vi "WPI_CANTalonSRX_ChangeMode.vi"(6 "Master Device Number":u8, 8 "error in (no error)":errorcluster, 9 "Output":dbl, 10 "Control Mode":T1=enum."Unchanged / Invalid", 11 "CAN Talon SRX Ref":T2={"DeviceStatus"={"status"=FALSE, "code"=0, "source"=""}, "Type"=enum."PWM", "PWM"={"PWM Channel"=enum."PWM 1", "DeadBand"={"Name"="", "maxPositivePwm"=0, "minPositivePwm"=0, "centerPwm"=0, "maxNegativePwm"=0, "minNegativePwm"=0, "angularRange"=0}}, "CAN"={"Device Number"=0, "SetOutput VI Ref"=variant(enum8{"Percent VBus", "Current", "Speed", "Position", "Voltage"} enum."Percent VBus"), "GetOutput VI Ref"=variant(refnum<k1> refnum), "Enable VI Ref"=variant(dbl 12.0), "Disable VI Ref"=variant(enum8{"Percent VBus", "Speed", "Position", "Slave", "Unchanged / Invalid", "Voltage Compensation", "Current", "Motion Profile"} enum."Percent VBus"), "Data"=variant}, "Invert"=FALSE}) -> (0 "error out":errorcluster, 3 "CAN Talon SRX Ref":T2={"DeviceStatus"={"status"=FALSE, "code"=0, "source"=""}, "Type"=enum."PWM", "PWM"={"PWM Channel"=enum."PWM 1", "DeadBand"={"Name"="", "maxPositivePwm"=0, "minPositivePwm"=0, "centerPwm"=0, "maxNegativePwm"=0, "minNegativePwm"=0, "angularRange"=0}}, "CAN"={"Device Number"=0, "SetOutput VI Ref"=variant(enum8{"Percent VBus", "Current", "Speed", "Position", "Voltage"} enum."Percent VBus"), "GetOutput VI Ref"=variant(refnum<k1> refnum), "Enable VI Ref"=variant(dbl 12.0), "Disable VI Ref"=variant(enum8{"Percent VBus", "Speed", "Position", "Slave", "Unchanged / Invalid", "Voltage Compensation", "Current", "Motion Profile"} enum."Percent VBus"), "Data"=variant}, "Invert"=FALSE})   [LabVIEW 2016]
doc: "Changes the Control Mode of the Talon SRX.\n\nYou must also set the output value when changing the mode.\n\n<B>Master Device Number</B> is the CAN bus device ID of the master controller and must be set if placing the current Talon SRX into \"Slave\" mode."
uses:
  <vilib>/Rock Robotics/WPI/MotorControl/WPI_MotorControlDeviceRef.ctl
  <vilib>/Rock Robotics/WPI/MotorControl/WPI_MotorControlType.ctl
  <vilib>/Rock Robotics/SystemInterfaces/DIO/FPGA_DIOPWMChannel.ctl
  <vilib>/Rock Robotics/WPI/PWM/WPI_PWMDeadband.ctl
  <vilib>/Rock Robotics/WPI/ThirdParty/CanMotor/TalonSRX/WPI_CANTalonSRX_APIControlMode.ctl
  <vilib>/Rock Robotics/WPI/ThirdParty/CanMotor/TalonSRX/WPI_CANTalonSRX_GlobalOps.ctl
  <vilib>/Rock Robotics/WPI/ThirdParty/CanMotor/TalonSRX/CTRE_CANTalonSRX_UsageTypes.ctl
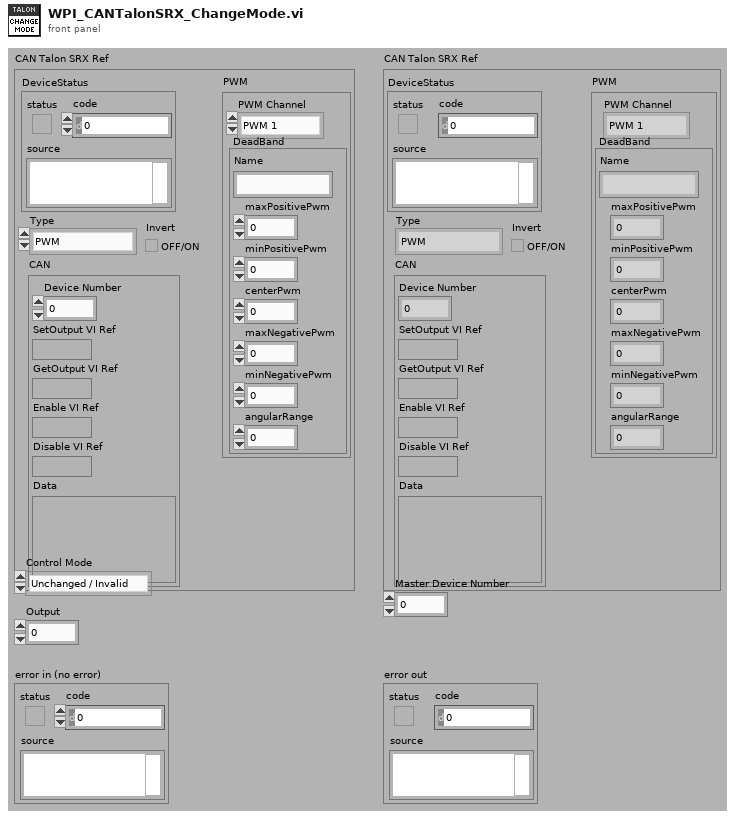
[diagram p1: front panel]
types:
  T1 = typedef "WPI_CANTalonSRX_APIControlMode.ctl" = enum8{"Percent VBus", "Speed", "Position", "Slave", "Unchanged / Invalid", "Voltage Compensation", "Current", "Motion Profile", "Motion Magic"}
  T2 = typedef "WPI_MotorControlDeviceRef.ctl" = cluster{"DeviceStatus":errorcluster, "Type":T3, "PWM":cluster{"PWM Channel":T4, "DeadBand":T5}, "CAN":cluster{"Device Number":u8, "SetOutput VI Ref":variant, "GetOutput VI Ref":variant, "Enable VI Ref":variant, "Disable VI Ref":variant, "Data":variant}, "Invert":bool}
  T3 = typedef "WPI_MotorControlType.ctl" = enum16{"PWM", "CAN"}
  T4 = typedef "FPGA_DIOPWMChannel.ctl" = enum8{"PWM 0", "PWM 1", "PWM 2", "PWM 3", "PWM 4", "PWM 5", "PWM 6", "PWM 7", "PWM 8", "PWM 9", "PWM MXP 0", "PWM MXP 1", "PWM MXP 2", "PWM MXP 3", "PWM MXP 4", "PWM MXP 5", "PWM MXP 6", "PWM MXP 7", "PWM MXP 8", "PWM MXP 9", "Invalid"}
  T5 = typedef "WPI_PWMDeadband.ctl" = cluster{"Name":string, "maxPositivePwm":i32, "minPositivePwm":i32, "centerPwm":i32, "maxNegativePwm":i32, "minNegativePwm":i32, "angularRange":u16}
  T6 = typedef "WPI_CANTalonSRX_GlobalOps.ctl" = enum16{"Read For Send", "Write After Receive General", "Write After Receive Feedback", "Write After Receive Encoder", "Write After Receive Ain", "Write Error", "Get All", "Set Output", "Set Mode", "Set Master ID", "Set Brake Mode", "Set Reverse Feedback Sensor", "Set Reverse Closed Loop Output", "Set Override Limits", "Set Forward Limit Enabled", "Set Reverse Limit Enabled", "Set Feedback Select", "Set Profile Select", "Set Throttle Ramp Rate", "Disable", "Set Enc Codes Per Rev", "Set Num Pot Turns", "Set Control Frame Rate", "Enable Legacy Control", "Write After Receive Pulse Width", "Set Enable Frame Rate", "Write After Receive Motion Profile", "Set Motion Profile Flow Control", "Set Motion Profile Control Frame Rate", "Set Current Limit Enable", "Set Usage Frame", "Write After Receive Motion Magic"}
  T7 = typedef "CTRE_CANTalonSRX_UsageTypes.ctl" = u32
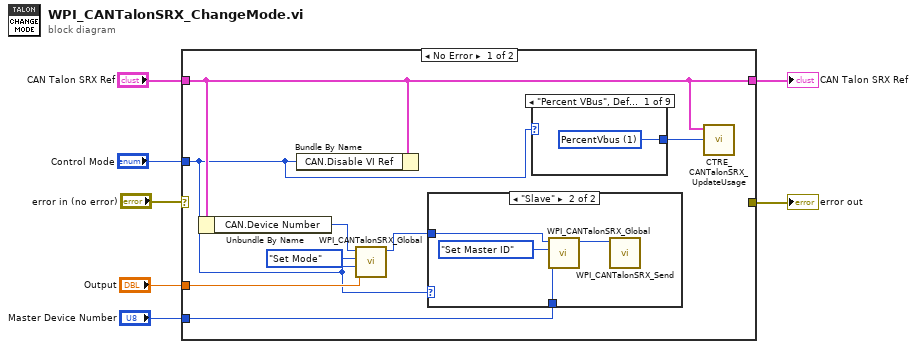
[diagram p0: block diagram]
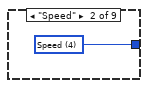
[diagram p2: hidden frame]
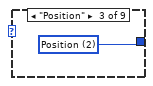
[diagram p3: hidden frame]
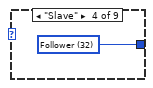
[diagram p4: hidden frame]
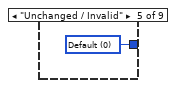
[diagram p5: hidden frame]
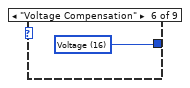
[diagram p6: hidden frame]
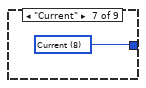
[diagram p7: hidden frame]
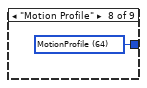
[diagram p8: hidden frame]
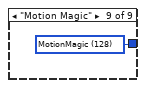
[diagram p9: hidden frame]
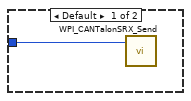
[diagram p10: hidden frame]
diagram:
  n1 = case shown="No Error" "error in (no error)" {
    selector: "error in (no error)" -> [_ w31]
    tunnel: [_ w31] -> w7
    tunnel: [w10 w30] -> w5
    tunnel: "CAN Talon SRX Ref" -> [w10 w30]
    tunnel: "Control Mode" -> [w8 _]
    tunnel: "Output" -> [w11 _]
    tunnel: "Master Device Number" -> [w12 _]
    frame No Error {
      n2 = Unbundle By Name(w10) -> ("CAN.Device Number"=w15:u8)
      n3 = Bundle By Name(cluster=w10, "CAN.Disable VI Ref"=w8) -> ()  [unwired: 1 out]
      n4 = call <vilib>:"WPI_CANTalonSRX_Global.vi"("Set Number"=w11, "Control Mode"=w8, "Operation"=WPI_CANTalonSRX_GlobalOps."Set Mode", "Device ID (0)"=w15) -> ("Device ID Out"=w13:u8)  [unwired: 5 in, 2 out]
      n5 = case shown="\"Slave\"" w8 {
        tunnel: w13 -> [w25 w28]
        tunnel: w12 -> [_ w27]
        frame Default {
          n6 = call <vilib>:"WPI_CANTalonSRX_Send.vi"("Device ID (0)"=w25) -> ()  [unwired: 10 in, 1 out]
        }
        frame "Slave" {
          n7 = call <vilib>:"WPI_CANTalonSRX_Global.vi"("Set Number"=w27, "Operation"=WPI_CANTalonSRX_GlobalOps."Set Master ID", "Device ID (0)"=w28) -> ("Device ID Out"=w26:u8)  [unwired: 6 in, 2 out]
          n8 = call <vilib>:"WPI_CANTalonSRX_Send.vi"("Device ID (0)"=w26) -> ()  [unwired: 10 in, 1 out]
        }
      }
      n9 = case shown="\"Percent VBus\", Default" w8 {
        tunnel: [w16 w17 w18 w19 w20 w21 w22 w23 w24] -> w9
        frame "Percent VBus", Default {
          w16 = T7 1 items=["Default"=0, "PercentVbus"=1, "Position"=2, "Speed"=4, "Current"=8, "Voltage"=16, "Follower"=32, "MotionProfile"=64, "MotionMagic"=128, "VRampRate"=4194304, "CurrentLimit"=8388608, "ZeroSensorI"=16777216, "ZeroSensorF"=33554432, "ZeroSensorR"=67108864, "ForwardLimitSwitch"=134217728, "ReverseLimitSwitch"=268435456, "ForwardSoftLimit"=536870912, "ReverseSoftLimit"=1073741824, "MultiProfile"=2147483648]
        }
        frame "Speed" {
          w17 = T7 4 items=["Default"=0, "PercentVbus"=1, "Position"=2, "Speed"=4, "Current"=8, "Voltage"=16, "Follower"=32, "MotionProfile"=64, "MotionMagic"=128, "VRampRate"=4194304, "CurrentLimit"=8388608, "ZeroSensorI"=16777216, "ZeroSensorF"=33554432, "ZeroSensorR"=67108864, "ForwardLimitSwitch"=134217728, "ReverseLimitSwitch"=268435456, "ForwardSoftLimit"=536870912, "ReverseSoftLimit"=1073741824, "MultiProfile"=2147483648]
        }
        frame "Position" {
          w18 = T7 2 items=["Default"=0, "PercentVbus"=1, "Position"=2, "Speed"=4, "Current"=8, "Voltage"=16, "Follower"=32, "MotionProfile"=64, "MotionMagic"=128, "VRampRate"=4194304, "CurrentLimit"=8388608, "ZeroSensorI"=16777216, "ZeroSensorF"=33554432, "ZeroSensorR"=67108864, "ForwardLimitSwitch"=134217728, "ReverseLimitSwitch"=268435456, "ForwardSoftLimit"=536870912, "ReverseSoftLimit"=1073741824, "MultiProfile"=2147483648]
        }
        frame "Slave" {
          w19 = T7 32 items=["Default"=0, "PercentVbus"=1, "Position"=2, "Speed"=4, "Current"=8, "Voltage"=16, "Follower"=32, "MotionProfile"=64, "MotionMagic"=128, "VRampRate"=4194304, "CurrentLimit"=8388608, "ZeroSensorI"=16777216, "ZeroSensorF"=33554432, "ZeroSensorR"=67108864, "ForwardLimitSwitch"=134217728, "ReverseLimitSwitch"=268435456, "ForwardSoftLimit"=536870912, "ReverseSoftLimit"=1073741824, "MultiProfile"=2147483648]
        }
        frame "Unchanged / Invalid" {
          w20 = T7 0 items=["Default"=0, "PercentVbus"=1, "Position"=2, "Speed"=4, "Current"=8, "Voltage"=16, "Follower"=32, "MotionProfile"=64, "MotionMagic"=128, "VRampRate"=4194304, "CurrentLimit"=8388608, "ZeroSensorI"=16777216, "ZeroSensorF"=33554432, "ZeroSensorR"=67108864, "ForwardLimitSwitch"=134217728, "ReverseLimitSwitch"=268435456, "ForwardSoftLimit"=536870912, "ReverseSoftLimit"=1073741824, "MultiProfile"=2147483648]
        }
        frame "Voltage Compensation" {
          w21 = T7 16 items=["Default"=0, "PercentVbus"=1, "Position"=2, "Speed"=4, "Current"=8, "Voltage"=16, "Follower"=32, "MotionProfile"=64, "MotionMagic"=128, "VRampRate"=4194304, "CurrentLimit"=8388608, "ZeroSensorI"=16777216, "ZeroSensorF"=33554432, "ZeroSensorR"=67108864, "ForwardLimitSwitch"=134217728, "ReverseLimitSwitch"=268435456, "ForwardSoftLimit"=536870912, "ReverseSoftLimit"=1073741824, "MultiProfile"=2147483648]
        }
        frame "Current" {
          w22 = T7 8 items=["Default"=0, "PercentVbus"=1, "Position"=2, "Speed"=4, "Current"=8, "Voltage"=16, "Follower"=32, "MotionProfile"=64, "MotionMagic"=128, "VRampRate"=4194304, "CurrentLimit"=8388608, "ZeroSensorI"=16777216, "ZeroSensorF"=33554432, "ZeroSensorR"=67108864, "ForwardLimitSwitch"=134217728, "ReverseLimitSwitch"=268435456, "ForwardSoftLimit"=536870912, "ReverseSoftLimit"=1073741824, "MultiProfile"=2147483648]
        }
        frame "Motion Profile" {
          w23 = T7 64 items=["Default"=0, "PercentVbus"=1, "Position"=2, "Speed"=4, "Current"=8, "Voltage"=16, "Follower"=32, "MotionProfile"=64, "MotionMagic"=128, "VRampRate"=4194304, "CurrentLimit"=8388608, "ZeroSensorI"=16777216, "ZeroSensorF"=33554432, "ZeroSensorR"=67108864, "ForwardLimitSwitch"=134217728, "ReverseLimitSwitch"=268435456, "ForwardSoftLimit"=536870912, "ReverseSoftLimit"=1073741824, "MultiProfile"=2147483648]
        }
        frame "Motion Magic" {
          w24 = T7 128 items=["Default"=0, "PercentVbus"=1, "Position"=2, "Speed"=4, "Current"=8, "Voltage"=16, "Follower"=32, "MotionProfile"=64, "MotionMagic"=128, "VRampRate"=4194304, "CurrentLimit"=8388608, "ZeroSensorI"=16777216, "ZeroSensorF"=33554432, "ZeroSensorR"=67108864, "ForwardLimitSwitch"=134217728, "ReverseLimitSwitch"=268435456, "ForwardSoftLimit"=536870912, "ReverseSoftLimit"=1073741824, "MultiProfile"=2147483648]
        }
      }
      n10 = call <vilib>:"CTRE_CANTalonSRX_UpdateUsage.vi"("Usage"=w9, "CAN Talon SRX Ref"=w10) -> ()  [unwired: 10 in]
    }
    frame Error {
    }
  }
  "CAN Talon SRX Ref" <- w5
  "error out" <- w7
